vi "VacuumSmoother.vi"(1 "Number Of Smooth Bins":i32, 2 "Newest Vacuum Sample":T1={"IG1 On"=TRUE, "IG2On"=FALSE, "IG Vac Level"=7.206095277894153e-07, "CG1 Vac Level"=7.188197481794052e-05, "CG2 Vac Level"=7.698533430214743e-05, "IG Status"=TRUE, "Turbo Gate"=FALSE} {"CG2 Vac Level" format="%#_2e"; "CG1 Vac Level" format="%#_2e"; "IG Vac Level" format="%#_2e"}, 3 "Vacuum Sample Smooth Cluster In":T2={"Vacuum Sample Array"=[], "Smoothed Vacuum Sample"={"IG1 On"=TRUE, "IG2On"=FALSE, "IG Vac Level"=7.206095277894153e-07, "CG1 Vac Level"=7.188197481794052e-05, "CG2 Vac Level"=7.698533430214743e-05, "IG Status"=TRUE, "Turbo Gate"=FALSE}} {"Smoothed Vacuum Sample"."CG2 Vac Level" format="%#_2e"; "Smoothed Vacuum Sample"."CG1 Vac Level" format="%#_2e"; "Smoothed Vacuum Sample"."IG Vac Level" format="%#_2e"; "Vacuum Sample Array"."CG2 Vac Level" format="%#_2e"; "Vacuum Sample Array"."CG1 Vac Level" format="%#_2e"; "Vacuum Sample Array"."IG Vac Level" format="%#_2e"}) -> (0 "Vacuum Sample Smooth Cluster Out":T2={"Vacuum Sample Array"=[], "Smoothed Vacuum Sample"={"IG1 On"=TRUE, "IG2On"=FALSE, "IG Vac Level"=7.206095277894153e-07, "CG1 Vac Level"=7.188197481794052e-05, "CG2 Vac Level"=7.698533430214743e-05, "IG Status"=TRUE, "Turbo Gate"=FALSE}} {"Smoothed Vacuum Sample"."CG2 Vac Level" format="%#_2e"; "Smoothed Vacuum Sample"."CG1 Vac Level" format="%#_2e"; "Smoothed Vacuum Sample"."IG Vac Level" format="%#_2e"; "Vacuum Sample Array"."CG2 Vac Level" format="%#_2e"; "Vacuum Sample Array"."CG1 Vac Level" format="%#_2e"; "Vacuum Sample Array"."IG Vac Level" format="%#_2e"})   [LabVIEW 2016]
uses:
  VacuumControls.ctl
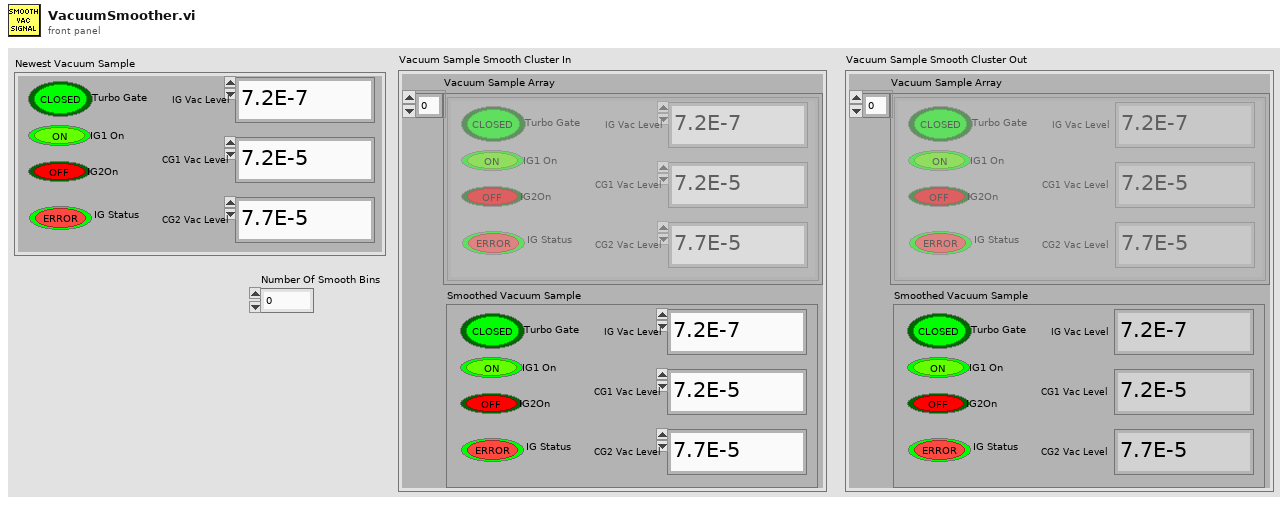
[diagram p1: front panel]
types:
  T1 = typedef "VacuumControls.ctl" = cluster{"IG1 On":bool, "IG2On":bool, "IG Vac Level":dbl, "CG1 Vac Level":dbl, "CG2 Vac Level":dbl, "IG Status":bool, "Turbo Gate":bool}
  T2 = cluster{"Vacuum Sample Array":T1[], "Smoothed Vacuum Sample":T1}
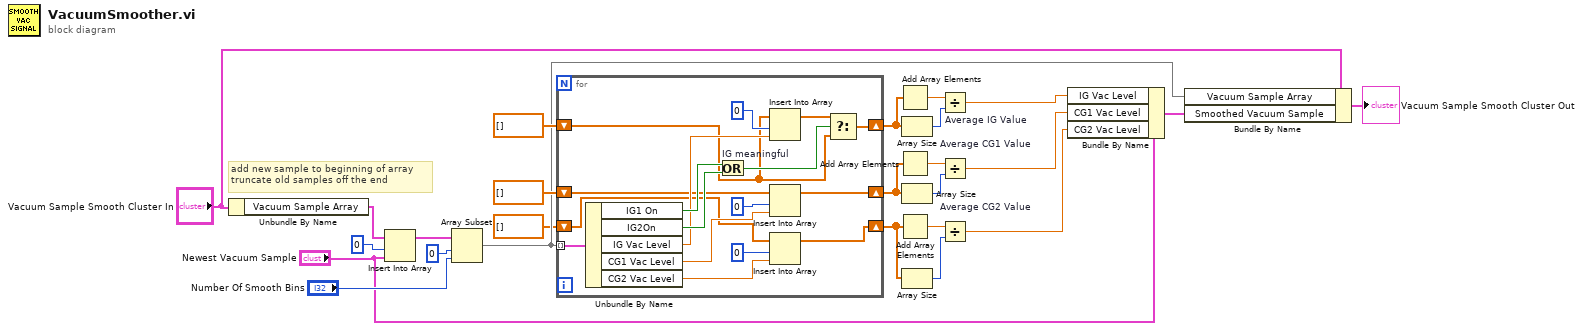
[diagram p0: block diagram]
diagram:
  # "add new sample to beginning of array\ntruncate old samples off the end"
  n1 = Unbundle By Name("Vacuum Sample Smooth Cluster In") -> ("Vacuum Sample Array"=w25:T1[])
  n2 = Insert Into Array(array=w25, index=0, new element="Newest Vacuum Sample") -> (w21:T1[])
  n3 = Array Subset(array=w21, index=0, length="Number Of Smooth Bins") -> (w8:T1[])
  n4 = for {
    tunnel: w8 -> [w42] mode=indexing
    shift-right: [w34] -> w16
    shift-left: dbl[] [] -> [w35]
    shift-right: [w30] -> w13
    shift-left: dbl[] [] -> [w32]
    shift-right: [w26] -> w2
    shift-left: dbl[] [] -> [w28]
    n5 = Unbundle By Name(w42) -> ("IG1 On"=w41:bool, "IG2On"=w40:bool, "IG Vac Level"=w37:dbl, "CG1 Vac Level"=w31:dbl, "CG2 Vac Level"=w27:dbl)
    n6 = Or "IG meaningful"(x=w41, y=w40) -> (x .or. y?=w39:bool)
    n7 = Insert Into Array(array=w35, index=0, new element=w37) -> (w36:dbl[])
    n8 = Insert Into Array(array=w32, index=0, new element=w31) -> (w30:dbl[])
    n9 = Insert Into Array(array=w28, index=0, new element=w27) -> (w26:dbl[])
    n10 = Select(t=w36, s=w39, f=w35) -> (s? t:f=w34:dbl[])
  }
  n11 = Add Array Elements(numeric array=w16) -> (sum=w18:dbl)
  n12 = Add Array Elements(numeric array=w13) -> (sum=w15:dbl)
  n13 = Add Array Elements(numeric array=w2) -> (sum=w4:dbl)
  n14 = Array Size(array=w16) -> (size(s)=w17:i32)
  n15 = Array Size(array=w13) -> (size(s)=w14:i32)
  n16 = Array Size(array=w2) -> (size(s)=w3:i32)
  n17 = Divide "Average IG Value"(x=w18, y=w17) -> (x/y=w12:dbl)
  n18 = Divide "Average CG1 Value"(x=w15, y=w14) -> (x/y=w11:dbl)
  n19 = Divide "Average CG2 Value"(x=w4, y=w3) -> (x/y=w1:dbl)
  n20 = Bundle By Name(cluster="Newest Vacuum Sample", "IG Vac Level"=w12, "CG1 Vac Level"=w11, "CG2 Vac Level"=w1) -> (w7:T1)
  n21 = Bundle By Name(cluster="Vacuum Sample Smooth Cluster In", "Vacuum Sample Array"=w8, "Smoothed Vacuum Sample"=w7) -> (→"Vacuum Sample Smooth Cluster Out":T2)
